vi "radnom spawn position.vi"() -> (3 "cluster of arrays of enemie data":cluster{dbl[], dbl[], dbl[]})   [LabVIEW 2019]
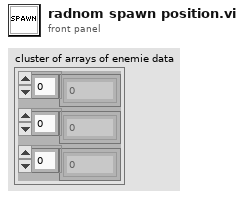
[diagram p1: front panel]
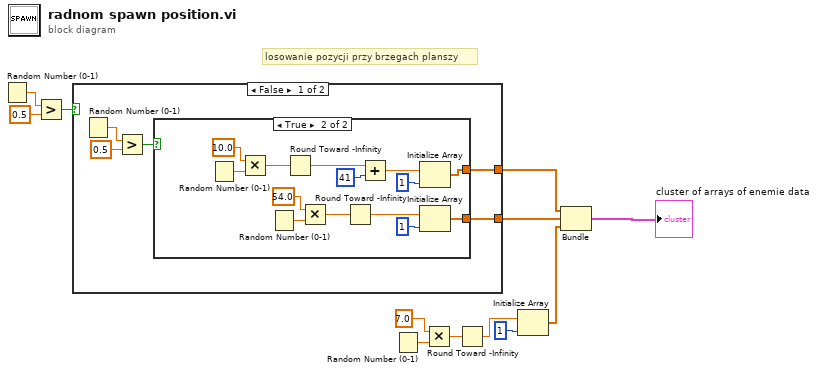
[diagram p0: block diagram]
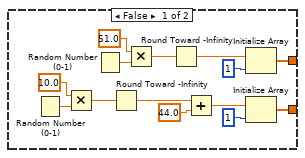
[diagram p2: hidden frame]
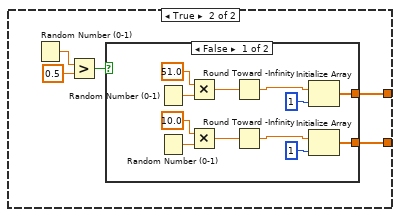
[diagram p3: hidden frame]
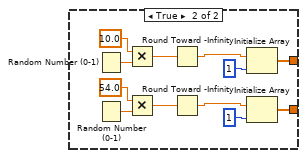
[diagram p4: hidden frame]
diagram:
  # "losowanie pozycji przy brzegach planszy"
  n1 = Random Number (0-1)() -> (number: 0 to 1=w11:dbl)
  n2 = Greater?(x=w11, y=0.5) -> (0:w12:bool)
  n3 = case shown="False" w12 {
    tunnel: [w14 w50] -> w3
    tunnel: [w13 w49] -> w4
    frame False {
      n4 = Random Number (0-1)() -> (number: 0 to 1=w17:dbl)
      n5 = Greater?(x=w17, y=0.5) -> (0:w15:bool)
      n6 = case shown="True" w15 {
        tunnel: [w22 w39] -> w14
        tunnel: [w21 w37] -> w13
        frame False {
          n7 = Random Number (0-1)() -> (number: 0 to 1=w26:dbl)
          n8 = Multiply(x=10.0, y=w26) -> (x*y=w31:dbl)
          n9 = Random Number (0-1)() -> (number: 0 to 1=w29:dbl)
          n10 = Round Toward -Infinity(1:w31) -> (0:w20:dbl)
          n11 = Multiply(x=51.0, y=w29) -> (x*y=w30:dbl)
          n12 = Round Toward -Infinity(1:w30) -> (0:w25:dbl)
          n13 = Add(x=w20, y=44.0) -> (x+y=w19:dbl)
          n14 = Initialize Array(w25, 1 ("dimension size")) -> (w22:dbl[])
          n15 = Initialize Array(w19, 1 ("dimension size")) -> (w21:dbl[])
        }
        frame True {
          n16 = Random Number (0-1)() -> (number: 0 to 1=w43:dbl)
          n17 = Multiply(x=10.0, y=w43) -> (x*y=w44:dbl)
          n18 = Random Number (0-1)() -> (number: 0 to 1=w40:dbl)
          n19 = Round Toward -Infinity(1:w44) -> (0:w33:dbl)
          n20 = Multiply(x=54.0, y=w40) -> (x*y=w45:dbl)
          n21 = Round Toward -Infinity(1:w45) -> (0:w38:dbl)
          n22 = Add(x=w33, y=41) -> (x+y=w32:dbl)
          n23 = Initialize Array(w32, 1 ("dimension size")) -> (w39:dbl[])
          n24 = Initialize Array(w38, 1 ("dimension size")) -> (w37:dbl[])
        }
      }
    }
    frame True {
      n25 = Random Number (0-1)() -> (number: 0 to 1=w48:dbl)
      n26 = Greater?(x=w48, y=0.5) -> (0:w46:bool)
      n27 = case shown="False" w46 {
        tunnel: [w52 w67] -> w50
        tunnel: [w51 w65] -> w49
        frame False {
          n28 = Random Number (0-1)() -> (number: 0 to 1=w60:dbl)
          n29 = Random Number (0-1)() -> (number: 0 to 1=w57:dbl)
          n30 = Multiply(x=51.0, y=w60) -> (x*y=w61:dbl)
          n31 = Multiply(x=10.0, y=w57) -> (x*y=w62:dbl)
          n32 = Round Toward -Infinity(1:w61) -> (0:w56:dbl)
          n33 = Round Toward -Infinity(1:w62) -> (0:w55:dbl)
          n34 = Initialize Array(w56, 1 ("dimension size")) -> (w52:dbl[])
          n35 = Initialize Array(w55, 1 ("dimension size")) -> (w51:dbl[])
        }
        frame True {
          n36 = Random Number (0-1)() -> (number: 0 to 1=w72:dbl)
          n37 = Random Number (0-1)() -> (number: 0 to 1=w69:dbl)
          n38 = Multiply(x=10.0, y=w72) -> (x*y=w73:dbl)
          n39 = Multiply(x=54.0, y=w69) -> (x*y=w74:dbl)
          n40 = Round Toward -Infinity(1:w73) -> (0:w68:dbl)
          n41 = Round Toward -Infinity(1:w74) -> (0:w66:dbl)
          n42 = Initialize Array(w68, 1 ("dimension size")) -> (w67:dbl[])
          n43 = Initialize Array(w66, 1 ("dimension size")) -> (w65:dbl[])
        }
      }
    }
  }
  n44 = Random Number (0-1)() -> (number: 0 to 1=w8:dbl)
  n45 = Multiply(x=7.0, y=w8) -> (x*y=w1:dbl)
  n46 = Round Toward -Infinity(1:w1) -> (0:w5:dbl)
  n47 = Initialize Array(w5, 1 ("dimension size")) -> (w6:dbl[])
  n48 = Bundle(w3, w4, w6) -> (→"cluster of arrays of enemie data":cluster{dbl[], dbl[], dbl[]})  [unwired: 1 in]
